vi "practice1.vi"() -> ()   [LabVIEW 2014]
uses:
  <vilib>/Motion/FlexMotion/CustomControls/CustomControls.llb/Axis To Control.flx
  <vilib>/Motion/FlexMotion/FunctionsVIs/StartStopMotion.llb/Start Motion (8 axes).flx
  <vilib>/Motion/FlexMotion/FunctionsVIs/Trajectory.llb/Check Move Complete Status (8 axes).flx
  <vilib>/Motion/FlexMotion/FunctionsVIs/StartStopMotion.llb/Stop Motion (8 axes).flx
  <instrlib>/KD Scientific 2XX Series/KD Scientific 2XX Series.lvlib
panel:
  in  "FIRST - Motor":bool
  out "Elapsed Time (s)":dbl format="%0.3f"
  in  "Motor speed\nmm/s":dbl
  in  "distance to move\nmm (post to post)":dbl
  out "Time from\nStart to finish (s)":dbl
  in  "stop 3":bool
  in  "stop 2":bool
  out "Voltage (V)":dbl=0.3869919147841388
  out "Force (grams)":dbl=0.3869919147841388
  out "Waveform Chart":dynamicdata(graph)
  in  "Zero":dbl=-99.6 format="%#_13g"
  out "Waveform Chart 2":dynamicdata(graph)
  in  "stop (F)":bool
  out "Data from Transducer":dynamicdata(graph) caption="data"
  out "Voltage from pressure transducer":dbl[](array[numeric])
  out "Pressure mm Hg":dbl[](graph)
  in  "Calibration factor":dbl[](array[numeric])
  in  "Zero Error":dbl[](array[numeric])
  out "pressure mm Hg":dbl[](array[numeric])
  in  "number of steps":i32
  out "Status":T1
  in  "stop":bool
  out "Delivered Volume":dbl
  out "Units":string
  in  "Baud Rate (9600)":u32(ring)=9600 items=["300"=300, "1200"=1200, "2400"=2400, "4800"=4800, "9600"=9600]
  in  "Withdrawal Settings":T2={"Flow Rate (5)"=5.0, "Volume (10)"=10.0, "Volume Units (ml)"=enum."milliliters (ml)", "Rate Units (ml/min.)"=enum."milliliters per minute (ml/min.)"} {"Volume (10)" format="%#.3g"}
  in  "Diameter (8.75 mm)":dbl=8.75
  in  "Infusion Settings":T2={"Flow Rate (5)"=5.0, "Volume (10)"=10.0, "Volume Units (ml)"=enum."milliliters (ml)", "Rate Units (ml/min.)"=enum."milliliters per minute (ml/min.)"}
  in  "Operation Mode (Infuse)":u16(ring) items=["Infuse", "Withdraw", "Infuse-Withdraw", "Withdraw-Infuse", "Continuous"]
  in  "Address (0)":i32 format="%0.0f"
  in  "error in (no error)":errorcluster
  in  "VISA resource name":refnum<visa-resource-name>="COM1"
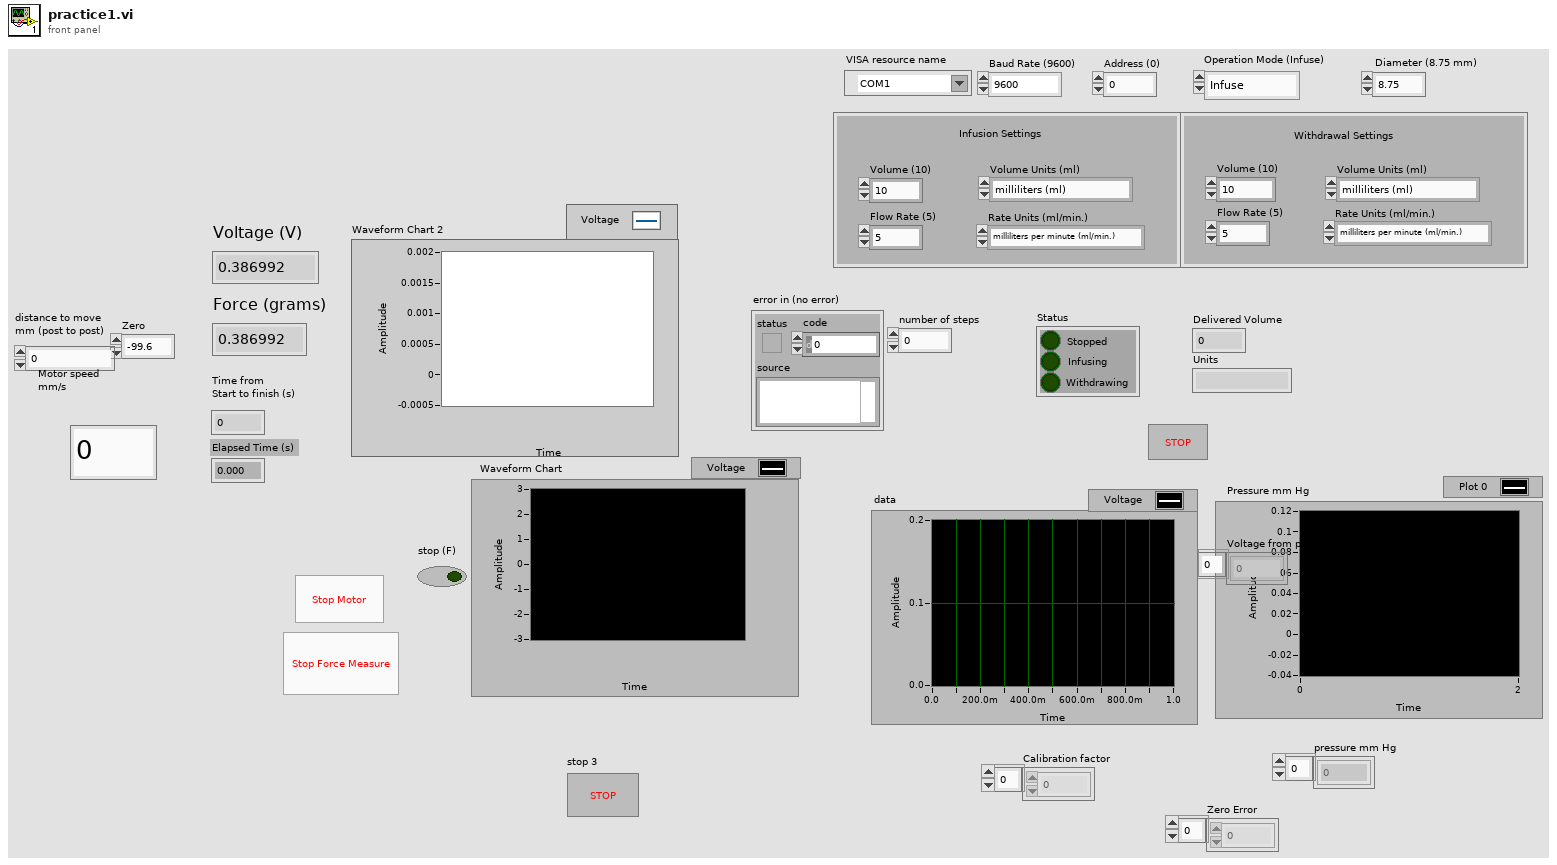
[diagram p1: front panel]
types:
  T1 = cluster{"Stopped":bool, "Infusing":bool, "Withdrawing":bool}
  T2 = cluster{"Flow Rate (5)":dbl, "Volume (10)":dbl, "Volume Units (ml)":enum16{"milliliters (ml)", "microliters (ul)"}, "Rate Units (ml/min.)":enum16{"milliliters per minute (ml/min.)", "milliliters per hour (ml/hr.)", "microliters per minute (ul/min.)", "microliters per hour (ul/hr.)"}}
  T3 = typedef "Board Id" = u8
  T4 = enum16{"Absolute Position", "Relative Position", "Velocity", "Relative to Cap Pos", "Modulus Position", "Absolute Contouring", "Relative Contouring"}
  T5 = typedef "Axis To Control.flx" = u16
  T6 = typedef "Resource Out (Enum).flx" = u16
  T7 = typedef "Bd Id Out" = u8
  T8 = enum16{"milliliters per minute (ml/min.)", "milliliters per hour (ml/hr.)", "microliters per minute (ul/min.)", "microliters per hour (ul/hr.)"}
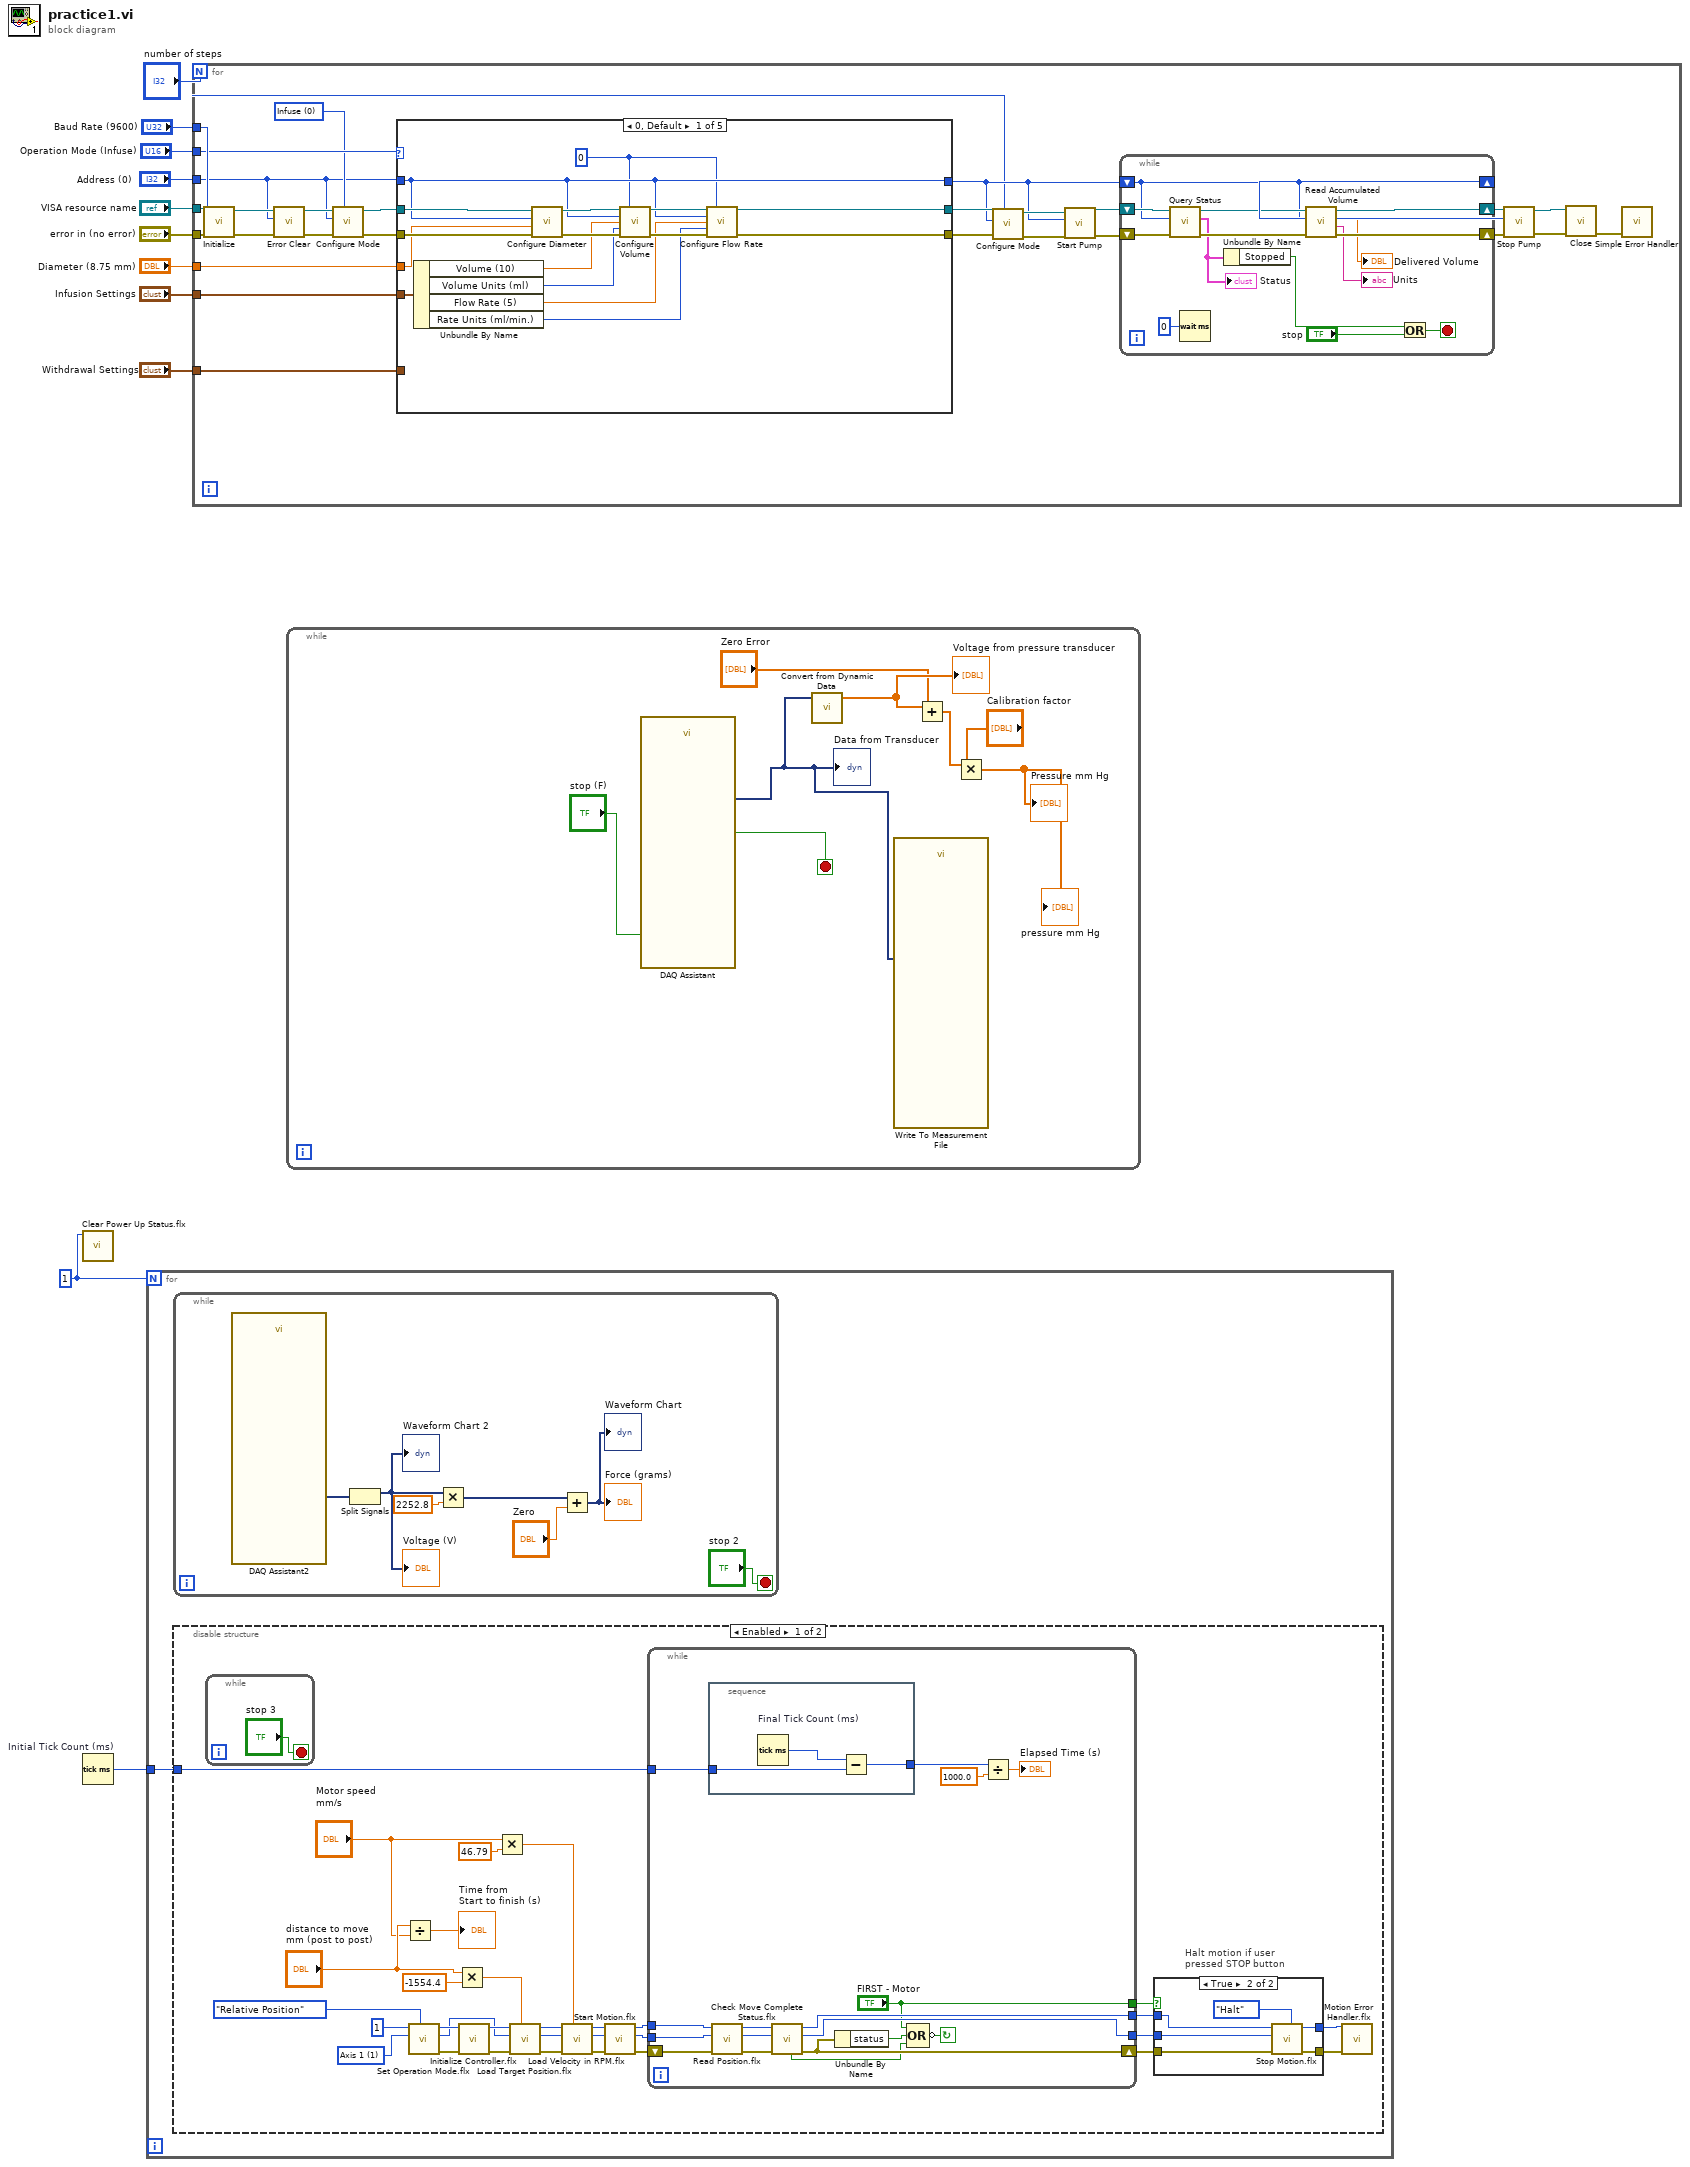
[diagram p0: block diagram]
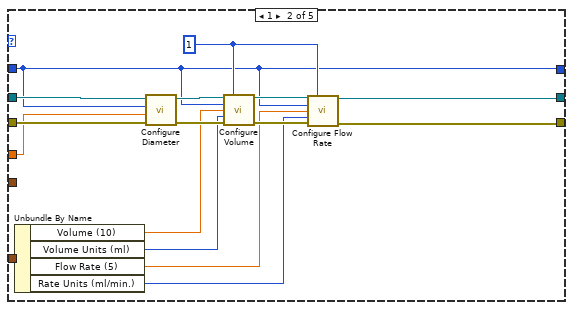
[diagram p4: hidden frame]
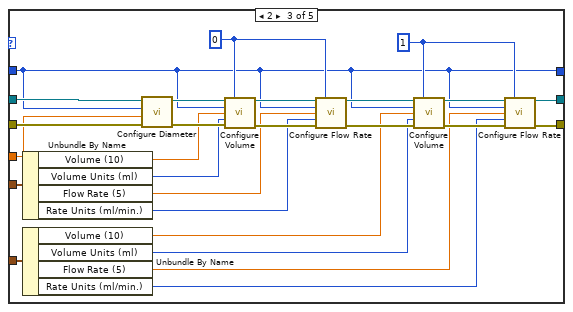
[diagram p5: hidden frame]
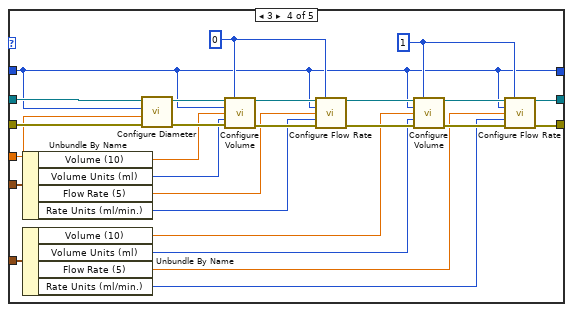
[diagram p6: hidden frame]
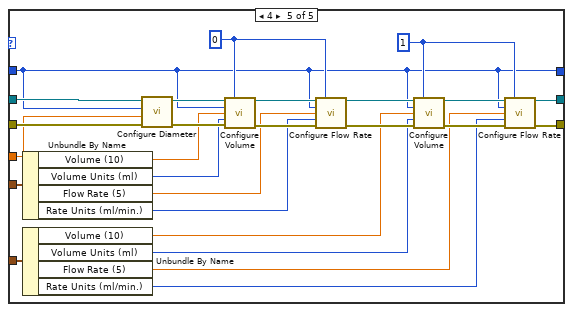
[diagram p7: hidden frame]
diagram:
  w2 = 1
  n1 = call <vilib>:"Clear Power Up Status.flx"("Board ID"=w2) -> ()  [unwired: 6 in, 2 out]
  n2 = Tick Count (ms) "Initial Tick Count (ms)"() -> (millisecond timer value=w1:u32)
  n3 = for {
    N: w2 -> [_]
    tunnel: w1 -> [w12]
    n4 = while {
      stop <- "stop 2" stop-if-true
      n5 = call "DAQ Assistant2"() -> ("data"=w18:dynamicdata)  [unwired: 16 in, 3 out]
      n6 = Split Signals(w18) -> (w13:dynamicdata)  [unwired: 2 in, 1 out]
      "Voltage (V)" <- w13
      "Waveform Chart 2" <- w13
      n7 = Multiply(x=w13, y=2252.8) -> (x*y=w17:dynamicdata)
      n8 = Add(x=w17, y="Zero") -> (x+y=→"Force (grams)" →"Waveform Chart":dynamicdata)
    }
    n9 = disable-structure shown="Enabled" {
      disable-tunnel: w12 -> [w23 _]
      frame Enabled {
        w40 = T5 1 items=["Axis 1"=1, "Axis 2"=2, "Axis 3"=3, "Axis 4"=4, "Axis 5"=5, "Axis 6"=6, "Axis 7"=7, "Axis 8"=8] ("Axis")
        # "Halt motion if user\npressed STOP button"
        n10 = while {
          stop <- "stop 3" stop-if-true
        }
        n11 = Divide(x="distance to move\nmm (post to post)", y="Motor speed\nmm/s") -> (x/y=→"Time from\nStart to finish (s)":dbl)
        n12 = call <vilib>:"Set Operation Mode.flx"("Position Mode (Absolute)"=T4."Relative Position", "Axis or Vector Space"=w40, "Board ID"=T3 1) -> ("error out"=w38:errorcluster, "Resource Output"=w20:T6, "Bd ID Out"=w37:T7)  [unwired: 3 in]
        n13 = Multiply(x="distance to move\nmm (post to post)", y=-1554.4) -> (x*y=w27:dbl)
        n14 = call <vilib>:"Initialize Controller.flx"("error in (no error)"=w38, "Board ID"=w37) -> ("error out"=w36:errorcluster, "Bd ID Out"=w35:T7)  [unwired: 6 in]
        n15 = Multiply(x="Motor speed\nmm/s", y=46.79) -> (x*y=w26:dbl)
        n16 = call <vilib>:"Load Target Position.flx"("Target Position (0)"=w27, "error in (no error)"=w36, "Axis"=w20, "Board ID"=w35) -> ("error out"=w48:errorcluster, "Resource Output"=w49:T6, "Bd ID Out"=w50:T7)  [unwired: 3 in]
        n17 = call <vilib>:"Load Velocity in RPM.flx"("Velocity (500)"=w26, "error in (no error)"=w48, "Axis or Vector Space"=w49, "Board ID"=w50) -> ("error out"=w41:errorcluster, "Resource Output"=w39:T6, "Bd ID Out"=w42:T7)  [unwired: 3 in]
        n18 = call-poly <vilib>:"Start Motion.flx"("error in (no error)"=w41, "Axis or Vector Space"=w39, "Board ID"=w42) -> ("error out"=w45:errorcluster, "Resource Output"=w44:T6, "Bd ID Out"=w43:T7)  [unwired: 3 in]
        n19 = while {
          tunnel: [w69] -> w29
          shift-left: w45 -> [w66]
          shift-right: [w70] -> w28
          tunnel: [w71] -> w30
          tunnel: w44 -> [w75]
          tunnel: w43 -> [w67]
          tunnel: w23 -> [w62]
          tunnel: ["FIRST - Motor"] -> w21
          stop <- w61 continue-if-true
          n20 = stacked-sequence {
            tunnel: w62 -> [w79]
            tunnel: [w77] -> w64
            frame #0 {
              n21 = Tick Count (ms) "Final Tick Count (ms)"() -> (millisecond timer value=w78:u32)
              n22 = Subtract(x=w78, y=w79) -> (x-y=w77:u32)
            }
          }
          n23 = call <vilib>:"Read Position.flx"("error in (no error)"=w66, "Axis"=w75, "Board ID"=w67) -> ("error out"=w73:errorcluster, "Resource Output"=w74:T6, "Bd ID Out"=w76:T7)  [unwired: 3 in, 1 out]
          n24 = call-poly <vilib>:"Check Move Complete Status.flx"("error in (no error)"=w73, "Axis or Vector Space"=w74, "Board ID"=w76) -> ("error out"=w70:errorcluster, "Resource Output"=w69:T6, "Bd ID Out"=w71:T7, "Move Complete"=w68:bool)  [unwired: 3 in]
          n25 = Unbundle By Name(w70) -> ("status"=w72:bool)
          n26 = Compound Arithmetic op=OR("FIRST - Motor", w72, w68) -> (invert w61:bool)
          n27 = Divide(x=w64, y=1000.0) -> (x/y=→"Elapsed Time (s)":dbl)
        }
        n28 = case shown="True" w21 {
          tunnel: w30 -> [w53 w58]
          tunnel: w28 -> [w52 w57]
          tunnel: [w52 w56] -> w34
          tunnel: [w53 w55] -> w33
          tunnel: w29 -> [_ w54]
          frame False {
          }
          frame True {
            n29 = call-poly <vilib>:"Stop Motion.flx"("Stop Type (Decel)"=enum16{"Decelerate", "Halt", "Kill"}."Halt", "error in (no error)"=w57, "Axis or Vector Space"=w54, "Board ID"=w58) -> ("error out"=w56:errorcluster, "Bd ID Out"=w55:T7)  [unwired: 3 in, 1 out]
          }
        }
        n30 = call <vilib>:"Motion Error Handler.flx"("Board ID"=w33, "error in (no error)"=w34) -> ()  [unwired: 9 in, 5 out]
      }
      frame Disabled {
      }
    }
  }
  n31 = for {
    N: "number of steps" -> [_]
    tunnel: "VISA resource name" -> [w107]
    tunnel: "error in (no error)" -> [w106]
    tunnel: "Infusion Settings" -> [w101]
    tunnel: "Withdrawal Settings" -> [w100]
    tunnel: "Diameter (8.75 mm)" -> [w99]
    tunnel: "Baud Rate (9600)" -> [w94]
    tunnel: "Operation Mode (Infuse)" -> [w88]
    tunnel: "Address (0)" -> [w80]
    w85 = u16 0 items=["Infuse", "Withdraw", "Infuse-Withdraw", "Withdraw-Infuse", "Continuous"] ("Mode (infuse)")
    n32 = call <instrlib>:"Initialize.vi"("error in (no error)"=w106, "Baud Rate (9600)"=w94, "VISA resource name"=w107) -> ("error out"=w82:errorcluster, "VISA resource name out"=w81:refnum<visa-resource-name>)  [unwired: 7 in]
    n33 = call <instrlib>:"Error Clear.vi"("error in (no error)"=w82, "Address (0)"=w80, "VISA resource name"=w81) -> ("error out"=w83:errorcluster, "VISA resource name out"=w84:refnum<visa-resource-name>)  [unwired: 6 in, 1 out]
    n34 = call <instrlib>:"Configure Mode.vi"("Mode (infuse)"=w85, "error in (no error)"=w83, "Address (0)"=w80, "VISA resource name"=w84) -> ("error out"=w87:errorcluster, "VISA resource name out"=w86:refnum<visa-resource-name>)  [unwired: 6 in]
    n35 = case shown="0, Default" w88 {
      tunnel: w101 -> [w117 _ w165 w191 w217]
      tunnel: w100 -> [_ w139 w164 w190 w216]
      tunnel: w86 -> [w123 w138 w163 w189 w215]
      tunnel: w87 -> [w122 w134 w162 w188 w214]
      tunnel: w99 -> [w116 w130 w145 w171 w197]
      tunnel: [w115 w124 w140 w166 w192] -> w89
      tunnel: w80 -> [w115 w124 w140 w166 w192]
      tunnel: [w110 w135 w142 w168 w194] -> w93
      tunnel: [w109 w131 w141 w167 w193] -> w92
      frame 0, Default {
        w108 = 0
        n36 = Unbundle By Name(w117) -> ("Volume (10)"=w114:dbl, "Volume Units (ml)"=w113:enum16{"milliliters (ml)", "microliters (ul)"}, "Flow Rate (5)"=w112:dbl, "Rate Units (ml/min.)"=w111:T8)
        n37 = call <instrlib>:"Configure Diameter.vi"("error in (no error)"=w122, "Diameter (8.75 mm)"=w116, "Address (0)"=w115, "VISA resource name"=w123) -> ("error out"=w120:errorcluster, "VISA resource name out"=w121:refnum<visa-resource-name>)  [unwired: 6 in]
        n38 = call <instrlib>:"Configure Volume.vi"("VISA resource name"=w121, "Mode (infuse)"=w108, "Address (0)"=w115, "Volume (100)"=w114, "Units (0: milliliters)"=w113, "error in (no error)"=w120) -> ("VISA resource name out"=w119:refnum<visa-resource-name>, "error out"=w118:errorcluster)  [unwired: 8 in]
        n39 = call <instrlib>:"Configure Flow Rate.vi"("VISA resource name"=w119, "Mode (infuse)"=w108, "Address (0)"=w115, "Flow Rate (5)"=w112, "Units (0: milliliters per minute)"=w111, "error in (no error)"=w118) -> ("VISA resource name out"=w110:refnum<visa-resource-name>, "error out"=w109:errorcluster)  [unwired: 8 in]
      }
      frame 1 {
        w125 = 1
        n40 = Unbundle By Name(w139) -> ("Volume (10)"=w129:dbl, "Volume Units (ml)"=w128:enum16{"milliliters (ml)", "microliters (ul)"}, "Flow Rate (5)"=w127:dbl, "Rate Units (ml/min.)"=w126:T8)
        n41 = call <instrlib>:"Configure Diameter.vi"("error in (no error)"=w134, "Diameter (8.75 mm)"=w130, "Address (0)"=w124, "VISA resource name"=w138) -> ("error out"=w133:errorcluster, "VISA resource name out"=w137:refnum<visa-resource-name>)  [unwired: 6 in]
        n42 = call <instrlib>:"Configure Volume.vi"("VISA resource name"=w137, "Mode (infuse)"=w125, "Address (0)"=w124, "Volume (100)"=w129, "Units (0: milliliters)"=w128, "error in (no error)"=w133) -> ("VISA resource name out"=w136:refnum<visa-resource-name>, "error out"=w132:errorcluster)  [unwired: 8 in]
        n43 = call <instrlib>:"Configure Flow Rate.vi"("VISA resource name"=w136, "Mode (infuse)"=w125, "Address (0)"=w124, "Flow Rate (5)"=w127, "Units (0: milliliters per minute)"=w126, "error in (no error)"=w132) -> ("VISA resource name out"=w135:refnum<visa-resource-name>, "error out"=w131:errorcluster)  [unwired: 8 in]
      }
      frame 2 {
        w143 = 1
        w144 = 0
        n44 = Unbundle By Name(w165) -> ("Volume (10)"=w153:dbl, "Volume Units (ml)"=w152:enum16{"milliliters (ml)", "microliters (ul)"}, "Flow Rate (5)"=w151:dbl, "Rate Units (ml/min.)"=w150:T8)
        n45 = Unbundle By Name(w164) -> ("Volume (10)"=w149:dbl, "Volume Units (ml)"=w148:enum16{"milliliters (ml)", "microliters (ul)"}, "Flow Rate (5)"=w147:dbl, "Rate Units (ml/min.)"=w146:T8)
        n46 = call <instrlib>:"Configure Diameter.vi"("error in (no error)"=w162, "Diameter (8.75 mm)"=w145, "Address (0)"=w140, "VISA resource name"=w163) -> ("error out"=w157:errorcluster, "VISA resource name out"=w161:refnum<visa-resource-name>)  [unwired: 6 in]
        n47 = call <instrlib>:"Configure Volume.vi"("VISA resource name"=w161, "Mode (infuse)"=w144, "Address (0)"=w140, "Volume (100)"=w153, "Units (0: milliliters)"=w152, "error in (no error)"=w157) -> ("VISA resource name out"=w160:refnum<visa-resource-name>, "error out"=w156:errorcluster)  [unwired: 8 in]
        n48 = call <instrlib>:"Configure Flow Rate.vi"("VISA resource name"=w160, "Mode (infuse)"=w144, "Address (0)"=w140, "Flow Rate (5)"=w151, "Units (0: milliliters per minute)"=w150, "error in (no error)"=w156) -> ("VISA resource name out"=w159:refnum<visa-resource-name>, "error out"=w155:errorcluster)  [unwired: 8 in]
        n49 = call <instrlib>:"Configure Volume.vi"("VISA resource name"=w159, "Mode (infuse)"=w143, "Address (0)"=w140, "Volume (100)"=w149, "Units (0: milliliters)"=w148, "error in (no error)"=w155) -> ("VISA resource name out"=w158:refnum<visa-resource-name>, "error out"=w154:errorcluster)  [unwired: 8 in]
        n50 = call <instrlib>:"Configure Flow Rate.vi"("VISA resource name"=w158, "Mode (infuse)"=w143, "Address (0)"=w140, "Flow Rate (5)"=w147, "Units (0: milliliters per minute)"=w146, "error in (no error)"=w154) -> ("VISA resource name out"=w142:refnum<visa-resource-name>, "error out"=w141:errorcluster)  [unwired: 8 in]
      }
      frame 3 {
        w169 = 1
        w170 = 0
        n51 = Unbundle By Name(w191) -> ("Volume (10)"=w179:dbl, "Volume Units (ml)"=w178:enum16{"milliliters (ml)", "microliters (ul)"}, "Flow Rate (5)"=w177:dbl, "Rate Units (ml/min.)"=w176:T8)
        n52 = Unbundle By Name(w190) -> ("Volume (10)"=w175:dbl, "Volume Units (ml)"=w174:enum16{"milliliters (ml)", "microliters (ul)"}, "Flow Rate (5)"=w173:dbl, "Rate Units (ml/min.)"=w172:T8)
        n53 = call <instrlib>:"Configure Diameter.vi"("error in (no error)"=w188, "Diameter (8.75 mm)"=w171, "Address (0)"=w166, "VISA resource name"=w189) -> ("error out"=w183:errorcluster, "VISA resource name out"=w187:refnum<visa-resource-name>)  [unwired: 6 in]
        n54 = call <instrlib>:"Configure Volume.vi"("VISA resource name"=w187, "Mode (infuse)"=w170, "Address (0)"=w166, "Volume (100)"=w179, "Units (0: milliliters)"=w178, "error in (no error)"=w183) -> ("VISA resource name out"=w186:refnum<visa-resource-name>, "error out"=w182:errorcluster)  [unwired: 8 in]
        n55 = call <instrlib>:"Configure Flow Rate.vi"("VISA resource name"=w186, "Mode (infuse)"=w170, "Address (0)"=w166, "Flow Rate (5)"=w177, "Units (0: milliliters per minute)"=w176, "error in (no error)"=w182) -> ("VISA resource name out"=w185:refnum<visa-resource-name>, "error out"=w181:errorcluster)  [unwired: 8 in]
        n56 = call <instrlib>:"Configure Volume.vi"("VISA resource name"=w185, "Mode (infuse)"=w169, "Address (0)"=w166, "Volume (100)"=w175, "Units (0: milliliters)"=w174, "error in (no error)"=w181) -> ("VISA resource name out"=w184:refnum<visa-resource-name>, "error out"=w180:errorcluster)  [unwired: 8 in]
        n57 = call <instrlib>:"Configure Flow Rate.vi"("VISA resource name"=w184, "Mode (infuse)"=w169, "Address (0)"=w166, "Flow Rate (5)"=w173, "Units (0: milliliters per minute)"=w172, "error in (no error)"=w180) -> ("VISA resource name out"=w168:refnum<visa-resource-name>, "error out"=w167:errorcluster)  [unwired: 8 in]
      }
      frame 4 {
        w195 = 1
        w196 = 0
        n58 = Unbundle By Name(w217) -> ("Volume (10)"=w205:dbl, "Volume Units (ml)"=w204:enum16{"milliliters (ml)", "microliters (ul)"}, "Flow Rate (5)"=w203:dbl, "Rate Units (ml/min.)"=w202:T8)
        n59 = Unbundle By Name(w216) -> ("Volume (10)"=w201:dbl, "Volume Units (ml)"=w200:enum16{"milliliters (ml)", "microliters (ul)"}, "Flow Rate (5)"=w199:dbl, "Rate Units (ml/min.)"=w198:T8)
        n60 = call <instrlib>:"Configure Diameter.vi"("error in (no error)"=w214, "Diameter (8.75 mm)"=w197, "Address (0)"=w192, "VISA resource name"=w215) -> ("error out"=w209:errorcluster, "VISA resource name out"=w213:refnum<visa-resource-name>)  [unwired: 6 in]
        n61 = call <instrlib>:"Configure Volume.vi"("VISA resource name"=w213, "Mode (infuse)"=w196, "Address (0)"=w192, "Volume (100)"=w205, "Units (0: milliliters)"=w204, "error in (no error)"=w209) -> ("VISA resource name out"=w212:refnum<visa-resource-name>, "error out"=w208:errorcluster)  [unwired: 8 in]
        n62 = call <instrlib>:"Configure Flow Rate.vi"("VISA resource name"=w212, "Mode (infuse)"=w196, "Address (0)"=w192, "Flow Rate (5)"=w203, "Units (0: milliliters per minute)"=w202, "error in (no error)"=w208) -> ("VISA resource name out"=w211:refnum<visa-resource-name>, "error out"=w207:errorcluster)  [unwired: 8 in]
        n63 = call <instrlib>:"Configure Volume.vi"("VISA resource name"=w211, "Mode (infuse)"=w195, "Address (0)"=w192, "Volume (100)"=w201, "Units (0: milliliters)"=w200, "error in (no error)"=w207) -> ("VISA resource name out"=w210:refnum<visa-resource-name>, "error out"=w206:errorcluster)  [unwired: 8 in]
        n64 = call <instrlib>:"Configure Flow Rate.vi"("VISA resource name"=w210, "Mode (infuse)"=w195, "Address (0)"=w192, "Flow Rate (5)"=w199, "Units (0: milliliters per minute)"=w198, "error in (no error)"=w206) -> ("VISA resource name out"=w194:refnum<visa-resource-name>, "error out"=w193:errorcluster)  [unwired: 8 in]
      }
    }
    n65 = call <instrlib>:"Configure Mode.vi"("Mode (infuse)"=w88, "error in (no error)"=w92, "Address (0)"=w89, "VISA resource name"=w93) -> ("error out"=w90:errorcluster, "VISA resource name out"=w91:refnum<visa-resource-name>)  [unwired: 6 in]
    n66 = call <instrlib>:"Start Pump.vi"("error in (no error)"=w90, "Address (0)"=w89, "VISA resource name"=w91) -> ("error out"=w104:errorcluster, "VISA resource name out"=w105:refnum<visa-resource-name>)  [unwired: 7 in]
    n67 = while {
      shift-right: [w220] -> w98
      shift-left: w89 -> [w220]
      shift-right: [w222] -> w103
      shift-left: w105 -> [w228]
      shift-right: [w221] -> w102
      shift-left: w104 -> [w229]
      stop <- w226 stop-if-true
      n68 = call <instrlib>:"Query Status.vi"("error in (no error)"=w229, "Address (0)"=w220, "VISA resource name"=w228) -> ("error out"=w231:errorcluster, "Status"=w227:T1, "VISA resource name out"=w223:refnum<visa-resource-name>)  [unwired: 6 in]
      "Status" <- w227
      n69 = Wait (ms)(milliseconds to wait=u32 0) -> ()  [unwired: 1 out]
      n70 = Unbundle By Name(w227) -> ("Stopped"=w225:bool)
      n71 = call <instrlib>:"Read Accumulated Volume.vi"("error in (no error)"=w231, "Address (0)"=w220, "VISA resource name"=w223) -> ("error out"=w221:errorcluster, "Units"=→"Units":string, "Delivered Volume"=→"Delivered Volume":dbl, "VISA resource name out"=w222:refnum<visa-resource-name>)  [unwired: 5 in]
      n72 = Or(x=w225, y="stop") -> (x .or. y?=w226:bool)
    }
    n73 = call <instrlib>:"Stop Pump.vi"("error in (no error)"=w102, "Address (0)"=w98, "VISA resource name"=w103) -> ("error out"=w96:errorcluster, "VISA resource name out"=w95:refnum<visa-resource-name>)  [unwired: 7 in]
    n74 = call <instrlib>:"Close.vi"("error in (no error)"=w96, "VISA resource name"=w95) -> ("error out"=w97:errorcluster)  [unwired: 9 in]
    n75 = call <vilib>:"Simple Error Handler.vi"("error in (no error)"=w97) -> ()  [unwired: 4 in, 5 out]
  }
  n76 = while {
    stop <- w238 stop-if-true
    n77 = call "DAQ Assistant"("stop (F)"="stop (F)") -> ("data"=w237:dynamicdata, "stopped"=w238:bool)  [unwired: 15 in, 2 out]
    "Data from Transducer" <- w237
    n78 = call "Convert from Dynamic Data"("Dynamic Data Type"=w237) -> ("Array"=w234:dbl[])  [unwired: 3 in]
    "Voltage from pressure transducer" <- w234
    n79 = call "Write To Measurement File"("Signals"=w237) -> ()  [unwired: 16 in, 3 out]
    n80 = Add(x=w234, y="Zero Error") -> (x+y=w232:dbl[])
    n81 = Multiply(x=w232, y="Calibration factor") -> (x*y=→"Pressure mm Hg" →"pressure mm Hg":dbl[])
  }
